vi "Construct.vi"(8 "Error in (no error)":errorcluster, 10 "Format":string="<logEntry>\n\t<timestamp>%Timestamp%</timestamp>\n\t<message>%Message%</message>\n\t<priority>%Priority%</priority>\n\t<priorityName>%PriorityName%</priorityName>\n</logEntry>") -> (0 "Error out":errorcluster, 3 "LogFormatterXml out":refnum<class "LogFormatterXml.lvclass">)   [LabVIEW 2011, in "LogFormatterXml.lvclass"]
uses:
  LogFormatterXml.lvclass
  LogFormatterXml.lvclass/LogFormatterXml.ctl
  LogFormatterSimple/LogFormatterSimple.lvclass
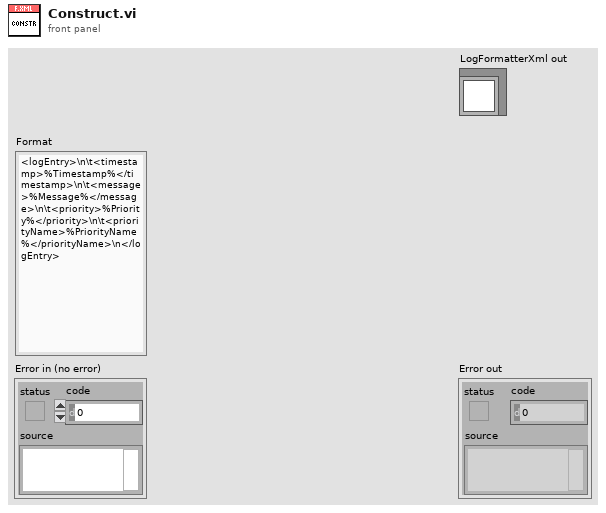
[diagram p1: front panel]
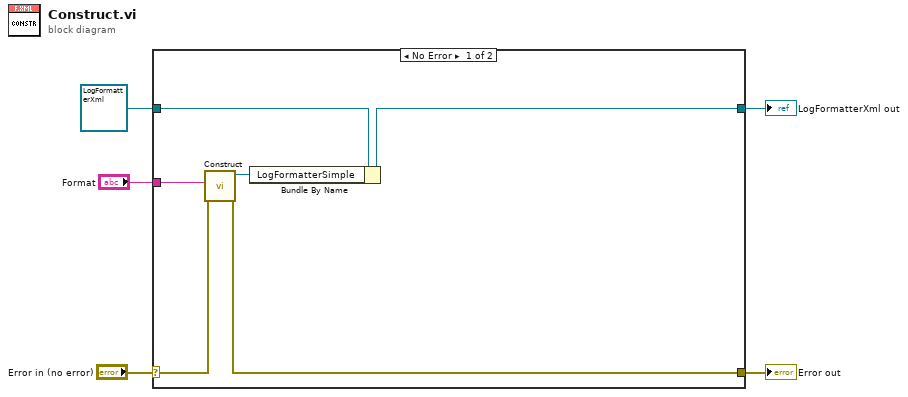
[diagram p0: block diagram]
diagram:
  n1 = case shown="No Error" "Error in (no error)" {
    selector: "Error in (no error)" -> [w10 w13]
    tunnel: [w9 w13] -> w4
    tunnel: [w6 w12] -> w3
    tunnel: refnum<class "LogFormatterXml.lvclass"> refnum ("LogFormatterXml in") -> [w7 w12]
    tunnel: "Format" -> [w11 _]
    frame No Error {
      n2 = call "Construct.vi"("Error in (no error)"=w10, "Format"=w11) -> ("Error out"=w9:errorcluster, "LogFormatterSimple out"=w8:refnum<class "LogFormatterSimple.lvclass">)  [unwired: 8 in]
      n3 = Bundle By Name(cluster=w7, "LogFormatterSimple"=w8) -> (w6:refnum<class "LogFormatterXml.lvclass">)
    }
    frame Error {
    }
  }
  "Error out" <- w4
  "LogFormatterXml out" <- w3
